vi "OE1311&OE1351_Data Index.vi"(1 "Parameter Type":u16(ring) items=["X", "Y", "R", "θ", "XD1", "YD1", "RD1", "θD1", "XD2", "YD2", "RD2", "θD2", "XD3", "YD3", "RD3", "θD3", "XD4", "YD4", "RD4", "θD4", "XD5", "YD5", "RD5", "θD5", "XD6", "YD6", "RD6", "θD6", "XD7", "YD7", "RD7", "θD7", "X_Noise", "Y_Noise", "Frequency", "AUX-IN1", "AUX-IN2"], 2 "Input Date Array":dbl[](array[numeric])) -> (0 "Parameter":dbl)   [LabVIEW 2011]
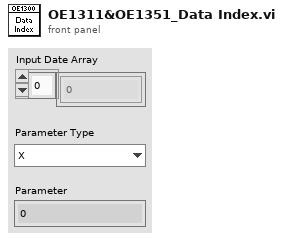
[diagram p1: front panel]
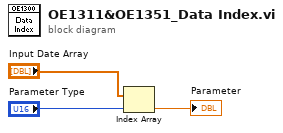
[diagram p0: block diagram]
diagram:
  n1 = Index Array(array="Input Date Array", index="Parameter Type") -> (element=→"Parameter":dbl)
